vi "subUnitCircle.vi"() -> (3 "XY Graph":cluster{"Y":dbl[], "Y":dbl[]}(graph))   [LabVIEW 2011]
panel:
  in  "Samples":i32=4001
  in  "Center":cdb
  in  "radius":dbl=1.0 format="%0.2p"
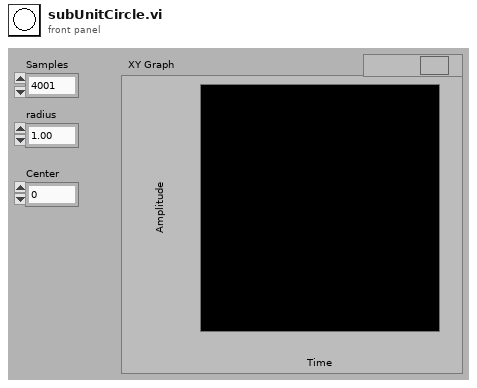
[diagram p1: front panel]
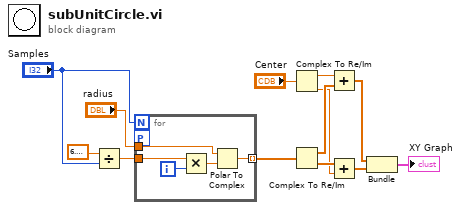
[diagram p0: block diagram]
diagram:
  n1 = Divide(x=6.283185307179586, y="Samples") -> (x/y=w9:dbl)
  n2 = for {
    N: "Samples" -> [_]
    tunnel: "radius" -> [w18]
    tunnel: w9 -> [w16]
    tunnel: [w14] -> w2 mode=indexing
    workers-P: _ -> [_]
    i -> [w17]
    n3 = Multiply(x=w16, y=w17) -> (x*y=w15:dbl)
    n4 = Polar To Complex(1:w15, 2:w18) -> (0:w14:cdb)
  }
  n5 = Complex To Re/Im(x + iy="Center") -> (x=w8:dbl, y=w4:dbl)
  n6 = Complex To Re/Im(x + iy=w2) -> (x=w7:dbl[], y=w5:dbl[])
  n7 = Add(x=w8, y=w7) -> (x+y=w6:dbl[])
  n8 = Add(x=w5, y=w4) -> (x+y=w3:dbl[])
  n9 = Bundle(w6, w3) -> (→"XY Graph":cluster{dbl[], dbl[]})  [unwired: 1 in]
